vi "Load Framework.vi"(8 "error in (no error)":errorcluster, 11 "Application Refs":T1={"Item Tree Control"=refnum, "Top-Level VI"=refnum, "menu reference"=refnum, "queue"=refnum, "Stop Pointer"=refnum, "Buffer Variant"=variant, "Framework Configuration"={"Plugins"=[]}, "server ID"=refnum, "framework tag"="", "Values"=refnum, "Hex"=refnum, "ASCII"=refnum, "lines visible"=0, "values padding"=0, "current buffer data"={"decimation"=0, "avg bandwidth"=-1.0, "channels"=[], "byte order"=enum."big-endian", "buffer descriptor"={"buffer type"=enum."Engine", "plugin id"=0, "group id"=0, "transfer id"=0, "offset"=0, "length"=0}, "values channels"={"index"=0, "count"=0, "engine offset"=0}, "select start offset"=18446744073709551615, "select end offset"=0}} {"current buffer data"."channels"."string offset" format="%d bytes"; "current buffer data"."avg bandwidth" format="%.0g bytes"}) -> (0 "error out":errorcluster, 3 "Application Data out":T1={"Item Tree Control"=refnum, "Top-Level VI"=refnum, "menu reference"=refnum, "queue"=refnum, "Stop Pointer"=refnum, "Buffer Variant"=variant, "Framework Configuration"={"Plugins"=[]}, "server ID"=refnum, "framework tag"="", "Values"=refnum, "Hex"=refnum, "ASCII"=refnum, "lines visible"=0, "values padding"=0, "current buffer data"={"decimation"=0, "avg bandwidth"=-1.0, "channels"=[], "byte order"=enum."big-endian", "buffer descriptor"={"buffer type"=enum."Engine", "plugin id"=0, "group id"=0, "transfer id"=0, "offset"=0, "length"=0}, "values channels"={"index"=0, "count"=0, "engine offset"=0}, "select start offset"=18446744073709551615, "select end offset"=0}} {"current buffer data"."channels"."string offset" format="%d bytes"; "current buffer data"."avg bandwidth" format="%.0g bytes"})   [LabVIEW 2017, in "DSF Core.lvlib"]
uses:
  DSF Core.lvlib
  Application Data.ctl
  Buffer Reader/Buffer Data.ctl
  <vilib>/NI/Memory Manager/Classes/Pointer/Pointer.lvclass
  Typedefs/DSF Timing Info.ctl
  Typedefs/DSF Settings Info.ctl
  Typedefs/DSF Engine Plugin Thread Configuration.ctl
  Typedefs/DSF Direction.ctl
  Typedefs/DSF Byte Order.ctl
  Typedefs/DSF Data Type.ctl
  Typedefs/DSF Engine Channel Configuration.ctl
  Typedefs/DSF Engine Transfer Configuration.ctl
  Typedefs/DSF Timeout Behavior.ctl
  Typedefs/DSF Engine Transfer Group Configuration.ctl
  Typedefs/DSF Engine Plugin Configuration.ctl
  Typedefs/DSF Engine Framework Configuration.ctl
  Typedefs/DSF Buffer Type.ctl
  Classes/Thread/Data Server/DSF Buffer Subset Descriptor.ctl
  Buffer Reader/Queue Data.ctl
  Values Channels.ctl
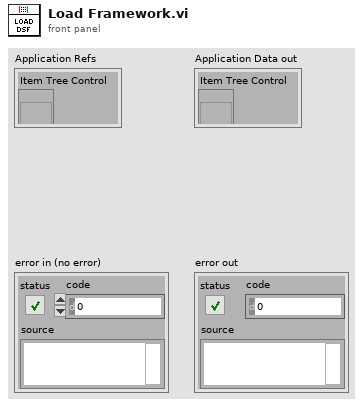
[diagram p1: front panel]
types:
  T1 = typedef "DSF Core.lvlib/Application Data.ctl" = cluster{"Item Tree Control":refnum<vi>, "Top-Level VI":refnum<vi>, "menu reference":refnum<k9>, "queue":refnum<queue>, "Stop Pointer":refnum<class "Pointer.lvclass">, "Buffer Variant":variant, "Framework Configuration":T2, "server ID":refnum<k5>, "framework tag":string, "Values":refnum<vi>, "Hex":refnum<vi>, "ASCII":refnum<vi>, "lines visible":i32, "values padding":i32, "current buffer data":T14}
  T2 = typedef "DSF Core.lvlib/DSF Engine Framework Configuration.ctl" = cluster{"Plugins":T3[]}
  T3 = typedef "DSF Core.lvlib/DSF Engine Plugin Configuration.ctl" = cluster{"name":string, "components":string[], "cycle timing":T4, "threads":T5[], "Transfer Groups":T7[], "settings":T6}
  T4 = typedef "DSF Core.lvlib/DSF Timing Info.ctl" = cluster{"priority":u64, "decimation":u64, "offset":u64}
  T5 = typedef "DSF Core.lvlib/DSF Engine Plugin Thread Configuration.ctl" = cluster{"buffer converter settings":T6, "transceiver settings":T6, "custom settings":T6, "processor":i32, "priority offset":i16}
  T6 = typedef "DSF Core.lvlib/DSF Settings Info.ctl" = cluster{"key":string, "value":string}[]
  T7 = typedef "DSF Core.lvlib/DSF Engine Transfer Group Configuration.ctl" = cluster{"name":string, "direction":T8, "cycle timing":T4, "thread index":i32, "settings":T6, "Transfers":T9[], "timeout behavior":T13}
  T8 = typedef "DSF Core.lvlib/DSF Direction.ctl" = enum8{"Tx", "Rx"}
  T9 = typedef "DSF Core.lvlib/DSF Engine Transfer Configuration.ctl" = cluster{"name":string, "byte order":T10, "settings":T6, "channels":T11[]}
  T10 = typedef "DSF Core.lvlib/DSF Byte Order.ctl" = enum8{"big-endian", "little-endian"}
  T11 = typedef "DSF Core.lvlib/DSF Engine Channel Configuration.ctl" = cluster{"string offset":u64, "string data type":T12, "engine data type":T12, "name":string, "settings":T6, "units":string}
  T12 = typedef "DSF Core.lvlib/DSF Data Type.ctl" = enum8{"Bool", "SGL", "DBL", "I8", "I16", "I32", "I64", "U8", "U16", "U32", "U64"}
  T13 = typedef "DSF Core.lvlib/DSF Timeout Behavior.ctl" = enum8{"Increment Late Count", "Throw Error"}
  T14 = typedef "DSF Core.lvlib/Buffer Data.ctl" = cluster{"decimation":u64, "avg bandwidth":dbl, "channels":T11[], "byte order":T10, "buffer descriptor":T15, "values channels":T17, "select start offset":u64, "select end offset":u64}
  T15 = typedef "DSF Core.lvlib/DSF Buffer Subset Descriptor.ctl" = cluster{"buffer type":T16, "plugin id":i32, "group id":i32, "transfer id":i32, "offset":u64, "length":i64}
  T16 = typedef "DSF Core.lvlib/DSF Buffer Type.ctl" = enum16{"Engine", "String"}
  T17 = typedef "DSF Core.lvlib/Values Channels.ctl" = cluster{"index":i32, "count":i32, "engine offset":u64}
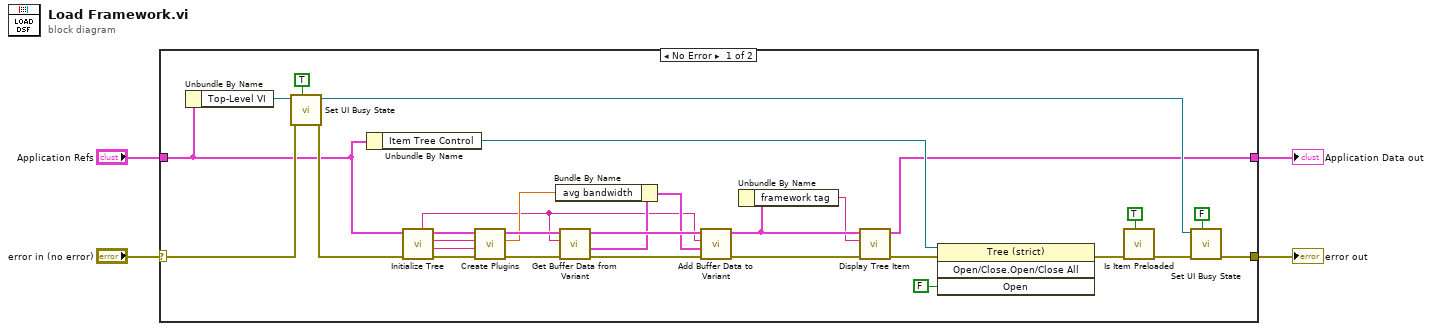
[diagram p0: block diagram]
diagram:
  n1 = case shown="No Error" "error in (no error)" {
    selector: "error in (no error)" -> [w13 w36]
    tunnel: [w7 w35] -> w4
    tunnel: [w14 w36] -> w3
    tunnel: "Application Refs" -> [w10 w35]
    frame No Error {
      n2 = Unbundle By Name(w10) -> ("Top-Level VI"=w19:refnum<vi>)
      n3 = call "Set UI Busy State.vi"("Defer Panel Updates"=TRUE, "error in (no error)"=w13, "VI in"=w19) -> ("error out"=w17:errorcluster, "VI out"=w12:refnum<vi>)  [unwired: 7 in]
      n4 = Unbundle By Name(w10) -> ("Item Tree Control"=w11:refnum<vi>)
      n5 = call "Initialize Tree.vi"("error in (no error)"=w17, "Application Data in"=w10) -> ("error out"=w32:errorcluster, "async plugins tag"=w30:string, "inline plugins tag"=w31:string, "Application Data out"=w33:T1, "framework tag"=w20:string)  [unwired: 5 in]
      n6 = call "Create Plugins.vi"("error in (no error)"=w32, "async plugins tag"=w30, "inline plugins tag"=w31, "Application Data In"=w33) -> ("error out"=w27:errorcluster, "avg bandwidth"=w22:dbl, "Application Data out"=w26:T1)  [unwired: 5 in]
      n7 = call "Get Buffer Data from Variant.vi"("error in (no error)"=w27, "tag"=w20, "Application Data In in"=w26) -> ("error out"=w24:errorcluster, "Buffer data"=w23:T14, "Application Data In out"=w25:T1)  [unwired: 6 in]
      n8 = Bundle By Name(cluster=w23, "avg bandwidth"=w22) -> (w21:T14)
      n9 = call "Add Buffer Data to Variant.vi"("error in (no error)"=w24, "Buffer data"=w21, "tag"=w20, "Application Data In in"=w25) -> ("error out"=w9:errorcluster, "Application Data In out"=w8:T1)  [unwired: 6 in]
      n10 = Unbundle By Name(w8) -> ("framework tag"=w5:string)
      n11 = call "Display Tree Item.vi"("error in (no error)"=w9, "Tag"=w5, "Application Data in"=w8) -> ("error out"=w6:errorcluster, "Application Data out"=w7:T1)  [unwired: 7 in]
      n12 = invoke class="Tree (strict)" method="Open/Close.Open/Close All"(reference=w11, error in=w6, "Open"=FALSE ("Open?")) -> (error out=w28:errorcluster)  [unwired: 1 in, 3 out]
      n13 = call "Is Item Preloaded"("clear entries"=TRUE, "error in (no error)"=w28) -> ("error out"=w15:errorcluster)  [unwired: 7 in, 2 out]
      n14 = call "Set UI Busy State.vi"("Defer Panel Updates"=FALSE, "error in (no error)"=w15, "VI in"=w12) -> ("error out"=w14:errorcluster)  [unwired: 7 in, 1 out]
    }
    frame Error {
    }
  }
  "error out" <- w3
  "Application Data out" <- w4
